vi "MultiPass_callback.vi"(7 "Method":enum16{"init", "run", "end"}(ring), 8 "error in (no error)":errorcluster, 10 "Pass":i32, 11 "Line":i32) -> (0 "error out":errorcluster)   [LabVIEW 2014]
doc: "Example Multipass scanning callback VI. Increases the bias voltage for each pass.\n\n- Nanonis Programming Interface -"
uses:
  <userlib>/Nanonis Prog Interface V5/Nanonis Prog Interface.lvlib
panel:
  in  "Override 2nd pass bias":bool
  in  "Bias (V) 2nd pass":sgl
  in  "Lockin ON/OFF":bool=TRUE
  in  "milliseconds to wait":u32=2
  in  "ref Bias (V)\nfirst pass":sgl=1.0 format="%_5p"
  # "this needs to be set \nin the first pass in the multipass panel"
  # "Callback VI connectors"
  # "Don't change the VI connector! Callback VIs must use the 4-2-2-4 connector pattern with these controls at the correct connectors to work!"
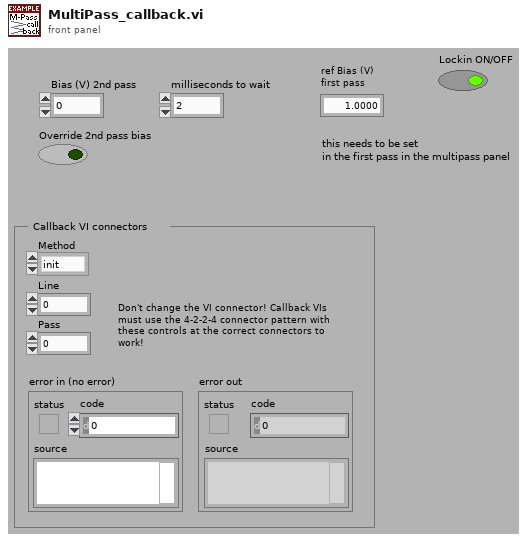
[diagram p1: front panel]
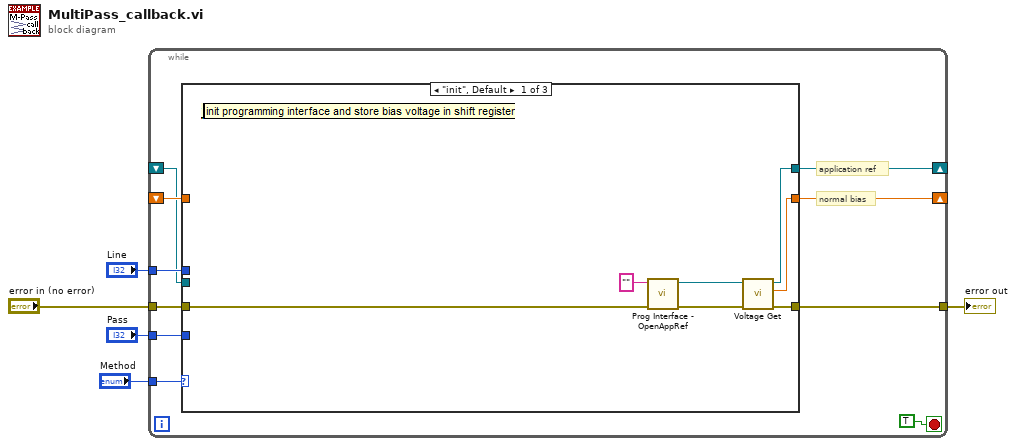
[diagram p0: block diagram]
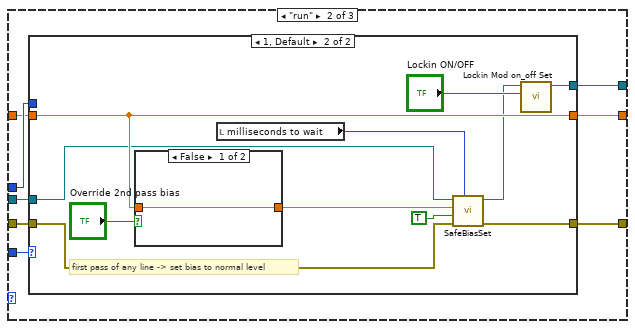
[diagram p2: hidden frame]
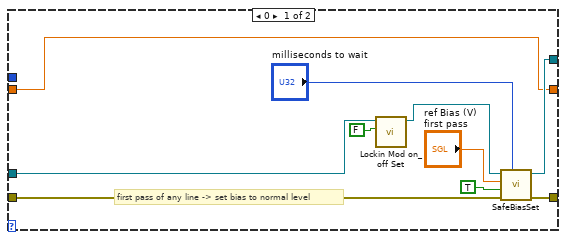
[diagram p3: hidden frame]
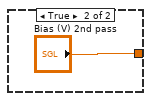
[diagram p4: hidden frame]
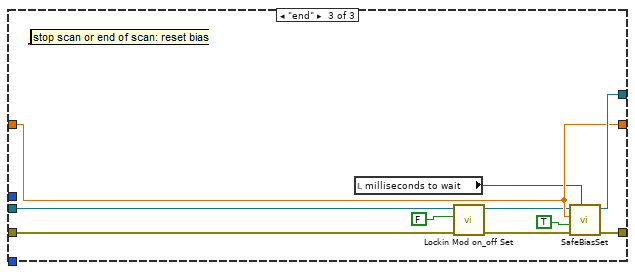
[diagram p5: hidden frame]
diagram:
  n1 = while {
    tunnel: "Pass" -> [w15]
    tunnel: "Line" -> [w14]
    tunnel: "error in (no error)" -> [w12]
    tunnel: [w13] -> w3
    shift-right: [w10] -> _
    shift-left: _ -> [w9]
    shift-right: [w8] -> _
    shift-left: _ -> [w7]
    tunnel: "Method" -> [w6]
    stop <- TRUE stop-if-true
    # "application ref"
    # "normal bias"
    n2 = case shown="\"init\", Default" w6 {
      tunnel: w15 -> [_ w30 _]
      tunnel: w14 -> [_ w29 _]
      tunnel: [w19 w28 w62] -> w13
      tunnel: w12 -> [w21 w27 w55]
      tunnel: [w18 w26 w61] -> w10
      tunnel: w9 -> [_ w25 w61]
      tunnel: [w16 w24 w63] -> w8
      tunnel: w7 -> [_ w23 w57]
      frame "init", Default {
        n3 = call <userlib>:"Prog Interface - OpenAppRef.vi"("Error in (no error)"=w21, "Machine name (local machine IP)"="") -> ("Error out"=w20:errorcluster, "Application reference"=w17:refnum<vi>)  [unwired: 4 in]
        n4 = call <userlib>:"Voltage Get.vi"("error in (no error)"=w20, "Application ref in"=w17) -> ("error out"=w19:errorcluster, "Bias (V)"=w18:sgl, "Application ref out"=w16:refnum<vi>)  [unwired: 7 in]
      }
      frame "run" {
        n5 = case shown="1, Default" w30 {
          tunnel: w29 -> [_ _]
          tunnel: [w38 w50] -> w28
          tunnel: w27 -> [w40 w51]
          tunnel: [w37 w45] -> w26
          tunnel: w25 -> [w37 w45]
          tunnel: [w39 w43] -> w24
          tunnel: w23 -> [w33 w42]
          frame 0 {
            # "first pass of any line -> set bias to normal level"
            n6 = call <userlib>:"Lockin Mod on_off Set.vi"("Lockin ON/OFF"=FALSE, "Application ref in"=w33) -> ("Application ref out"=w32:refnum<vi>)  [unwired: 8 in, 1 out]
            n7 = call "SafeBiasSet.vi"("Application ref in"=w32, "Bias (V)"="ref Bias (V)\nfirst pass", "Ramp"=TRUE, "error in (no error)"=w40, "milliseconds to wait"="milliseconds to wait") -> ("Application ref out"=w39:refnum<vi>, "Error out"=w38:errorcluster)  [unwired: 4 in]
          }
          frame 1, Default {
            # "first pass of any line -> set bias to normal level"
            n8 = case shown="False" "Override 2nd pass bias" {
              tunnel: [w52 "Bias (V) 2nd pass"] -> w46
              tunnel: w45 -> [w52 _]
              frame False {
              }
              frame True {
              }
            }
            n9 = local read "milliseconds to wait"() -> (w48:u32)
            n10 = call "SafeBiasSet.vi"("Application ref in"=w42, "Bias (V)"=w46, "Ramp"=TRUE, "error in (no error)"=w51, "milliseconds to wait"=w48) -> ("Application ref out"=w41:refnum<vi>, "Error out"=w50:errorcluster)  [unwired: 4 in]
            n11 = call <userlib>:"Lockin Mod on_off Set.vi"("Lockin ON/OFF"="Lockin ON/OFF", "Application ref in"=w41) -> ("Application ref out"=w43:refnum<vi>)  [unwired: 8 in, 1 out]
          }
        }
      }
      frame "end" {
        n12 = local read "milliseconds to wait"() -> (w60:u32)
        n13 = call <userlib>:"Lockin Mod on_off Set.vi"("Error in (no error)"=w55, "Lockin ON/OFF"=FALSE, "Application ref in"=w57) -> ("Error out"=w54:errorcluster, "Application ref out"=w56:refnum<vi>)  [unwired: 7 in]
        n14 = call "SafeBiasSet.vi"("Application ref in"=w56, "Bias (V)"=w61, "Ramp"=TRUE, "error in (no error)"=w54, "milliseconds to wait"=w60) -> ("Application ref out"=w63:refnum<vi>, "Error out"=w62:errorcluster)  [unwired: 4 in]
      }
    }
  }
  "error out" <- w3
